vi "formula node.vi"() -> ()   [LabVIEW 2012]
panel:
  out "L":dbl
  out "A":dbl
  out "Z":dbl
  in  "Y":dbl
  in  "X":dbl
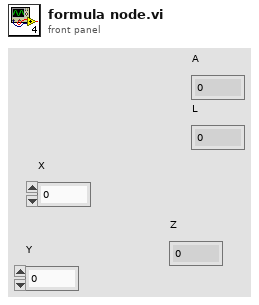
[diagram p1: front panel]
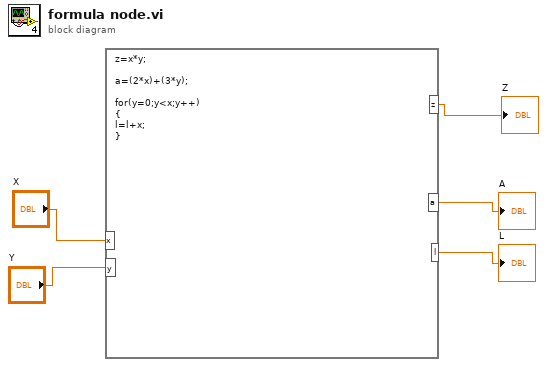
[diagram p0: block diagram]
diagram:
  n1 = formula code="z=x*y;\n\na=(2*x)+(3*y);\n\nfor(y=0;y<x;y++)\n{\nl=l+x;\n}"("x"="X", "y"="Y") -> ("z"=→"Z":dbl, "a"=→"A":dbl, "l"=→"L":dbl)
